vi "Wait For N Elements Available.vi"(8 "Error in":errorcluster, 9 "N Elements":u32=1, 10 "Timeout (ns)":i64, 11 "CIPC Reference":u64) -> (0 "Error out":errorcluster, 1 "Time Out":bool, 2 "Time Remaining (ns)":i64)   [LabVIEW 2021, in "CIF_NI_CIPC.lvlib"]
doc: "Wait until the N elements, starting from the current reading location, are written by the CIPC writer."
uses:
  CIF_NI_CIPC.lvlib
  <vilib>/Utility/error.llb/Trim Whitespace.vi
  <vilib>/Utility/error.llb/Error Cluster From Error Code.vi
  libnicipc.dll
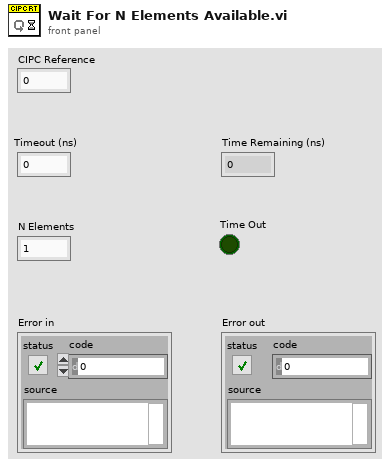
[diagram p1: front panel]
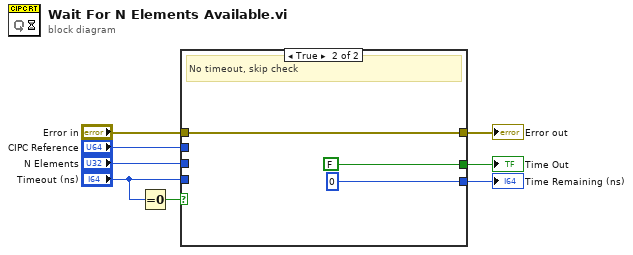
[diagram p0: block diagram]
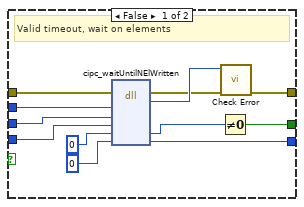
[diagram p2: hidden frame]
diagram:
  n1 = Equal To 0?(x="Timeout (ns)") -> (x = 0?=w1:bool)
  n2 = case shown="True" w1 {
    tunnel: [w18 w23] -> w8
    tunnel: "Timeout (ns)" -> [w17 _]
    tunnel: [w15 i64 0 ("time_left")] -> w7
    tunnel: [w12 FALSE] -> w6
    tunnel: "Error in" -> [w11 w23]
    tunnel: "N Elements" -> [w10 _]
    tunnel: "CIPC Reference" -> [w9 _]
    frame False {
      # "Valid timeout, wait on elements"
      n3 = dll-call lib="libnicipc.*" fn="cipc_waitUntilNElWritten"(error in=w11, "cipc_buffer_ref"=w9, "N"=w10, "timeout_ns"=w17, "timed_out"=u8 0 ("timeout_ns"), "time_left"=i64 0 ("timeout_ns")) -> (error out=w19:errorcluster, "return type"=w20:i32, "timed_out"=w13:u8, "time_left"=w15:i64)  [unwired: 5 in, 1 out]
      n4 = Not Equal To 0?(x=w13) -> (x != 0?=w12:bool)
      n5 = call "Check Error.vi"("error in (no error)"=w19, "Error Code"=w20) -> ("error out"=w18:errorcluster)  [unwired: 9 in]
    }
    frame True {
      # "No timeout, skip check"
    }
  }
  "Error out" <- w8
  "Time Out" <- w6
  "Time Remaining (ns)" <- w7
